vi "New Verify CLI Output.vi"   [LabVIEW 2020, in "Caraya.Extension.lvlib"]
uses:
  Caraya.Extension.lvlib
  <vilib>/addons/_JKI Toolkits/Caraya/classes/Test/Test.lvclass
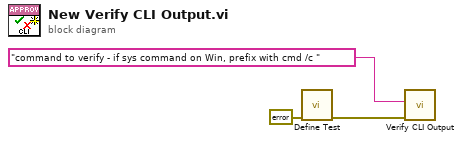
[diagram p0: block diagram]
diagram:
  n1 = call <vilib>:"Define Test.vi"("error in (no error)"=errorcluster {"status"=FALSE, "code"=0, "source"=""}) -> ("error out"=w2:errorcluster)  [unwired: 9 in, 1 out]
  n2 = call "Verify CLI Output.vi"("error in"=w2, "command line"="command to verify - if sys command on Win, prefix with cmd /c ") -> ()  [unwired: 8 in, 2 out]
